vi "TcpServer.vi"(4 "WriteTimeout [ms] (5000)":i32=5000, 5 "ConnectionTimeout [ms] (5000)":i32=5000, 6 "ReadTimeout [ms] (5000)":i32=5000, 7 "ReadMode (Standard)":T1(ring), 8 "error in (no error)":errorcluster, 9 "OpenTimeout [ms] (5000)":i32=5000, 10 "Port in (0)":u16, 11 "IpAddress (127.0.0.1)":string="127.0.0.1") -> (0 "error out":errorcluster, 2 "Port out":u16, 3 "TcpServer":refnum<class "TcpServer.lvclass">)   [LabVIEW 2021, in "TcpServer.lvlib" / "TcpServer.lvclass"]
uses:
  TcpServer.lvclass
  D:/_uliarczj/LabVIEW/LvTcpSocket/LvTcpSocket/Source/TcpSocket/TcpSocket/TcpSocket.lvclass
  TcpSocket/TcpSocket/TcpSocket.lvclass/TcpSocket.ctl
  TcpServer.lvclass/TcpServer.ctl
  TcpSocket/TcpSocket/Write ReadMode.vi
  TcpSocket/TcpSocket/Write Address.vi
  TcpSocket/TcpSocket/Write Connection.vi
  TcpSocket/TcpSocket/Write Port.vi
  TcpSocket/TcpSocket/Write OpenTimeout.vi
  TcpSocket/TcpSocket/Write ReadTimeout.vi
  TcpSocket/TcpSocket/Write WriteTimeout.vi
  Write ConnectionTimeout.vi
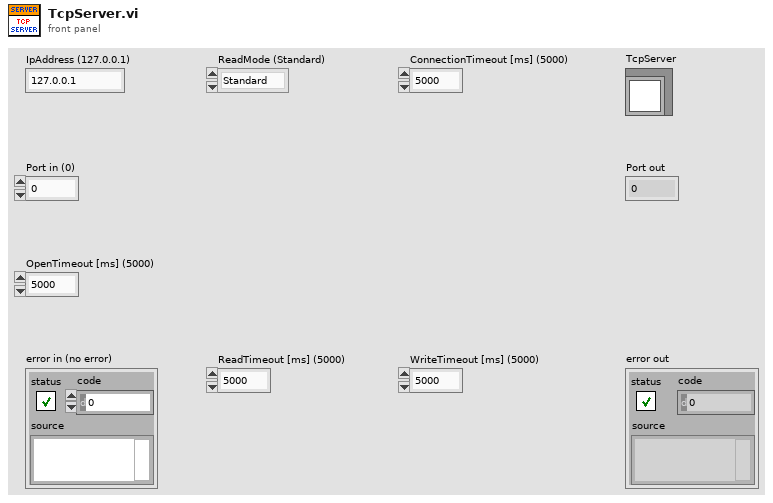
[diagram p1: front panel]
types:
  T1 = enum16{"Standard", "Buffered", "CRLF", "Immediate"}
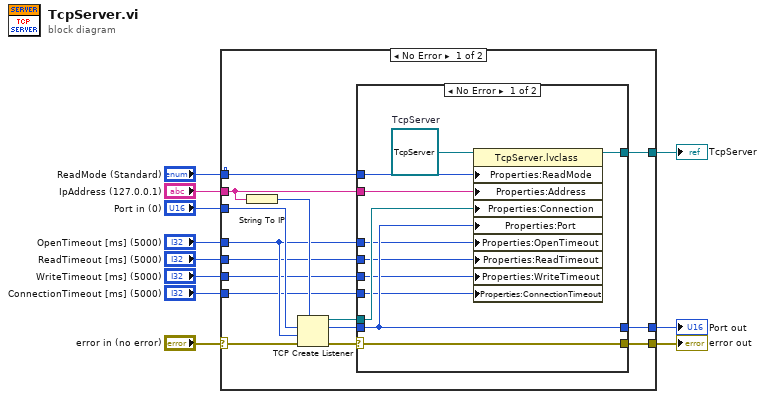
[diagram p0: block diagram]
diagram:
  n1 = case shown="No Error" "error in (no error)" {
    selector: "error in (no error)" -> [w26 w39]
    tunnel: [w23 w39] -> w10
    tunnel: [w22 _] -> w9
    tunnel: "Port in (0)" -> [w21 _]
    tunnel: "IpAddress (127.0.0.1)" -> [w20 _]
    tunnel: "OpenTimeout [ms] (5000)" -> [w17 _]
    tunnel: "ReadMode (Standard)" -> [w16 _]
    tunnel: "ConnectionTimeout [ms] (5000)" -> [w15 _]
    tunnel: "ReadTimeout [ms] (5000)" -> [w14 _]
    tunnel: [w13 _] -> w2
    tunnel: "WriteTimeout [ms] (5000)" -> [w12 _]
    frame No Error {
      n2 = String To IP(1:w20) -> (0:w25:u32)
      n3 = TCP Create Listener(7:w25, 8:w26, 9:w17, 10:w21) -> (0:w24:errorcluster, 2:w18:u16, 3:w19:refnum<k5>)  [unwired: 1 in]
      n4 = case shown="No Error" w24 {
        selector: w24 -> [w37 w38]
        tunnel: [w37 w38] -> w23
        tunnel: [w35 _] -> w22
        tunnel: w20 -> [w33 _]
        tunnel: w19 -> [w32 _]
        tunnel: w18 -> [w31 _]
        tunnel: w17 -> [w30 _]
        tunnel: w16 -> [w34 _]
        tunnel: w15 -> [w28 _]
        tunnel: w14 -> [w29 _]
        tunnel: [w31 _] -> w13
        tunnel: w12 -> [w27 _]
        frame No Error {
          w36 = refnum<class "TcpServer.lvclass"> refnum  # TcpServer
          n5 = property class="TcpServer.lvclass"(reference=w36, "Properties:ReadMode"=w34, "Properties:Address"=w33, "Properties:Connection"=w32, "Properties:Port"=w31, "Properties:OpenTimeout"=w30, "Properties:ReadTimeout"=w29, "Properties:WriteTimeout"=w27, "Properties:ConnectionTimeout"=w28) -> (reference out=w35:refnum<class "TcpServer.lvclass">)  [unwired: 1 in, 1 out]
        }
        frame Error {
        }
      }
    }
    frame Error {
    }
  }
  "error out" <- w10
  "TcpServer" <- w9
  "Port out" <- w2
